vi "Build Command.vi"(8 "Error In":errorcluster, 9 "Field Data":u8[](array[numeric]) format="%02x", 10 "Field Descriptor Byte":u8=117 format="%02x", 11 "Data Set":T1=enum."NAV") -> (0 "Error Out":errorcluster, 3 "Command":u8[](array[numeric]) format="%02x")   [LabVIEW 2011]
doc: "This VI builds Hex commands for the Microstrain 3DM GX3-45 \n\nSee Microstrain Communications Protocol guide for further details."
uses:
  Controls/Desciptor Set Byte.ctl
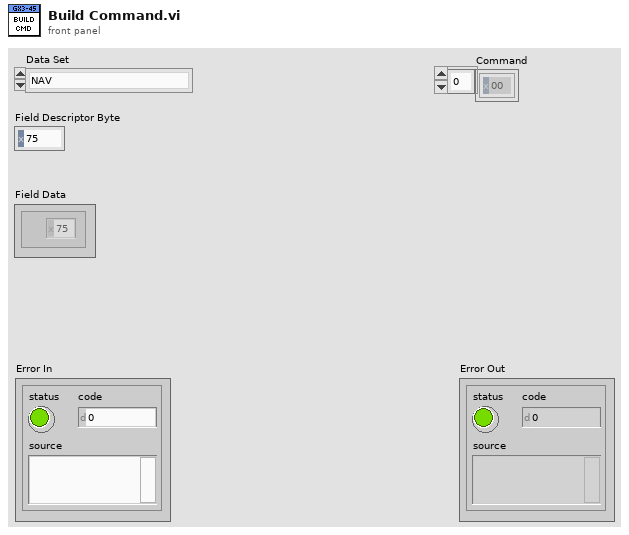
[diagram p1: front panel]
types:
  T1 = typedef "Desciptor Set Byte.ctl" = enum16{"Base Command Set", "3DM Command Set", "Navigation Filter Command Set", "System Command Set", "AHRS", "GPS", "NAV"}
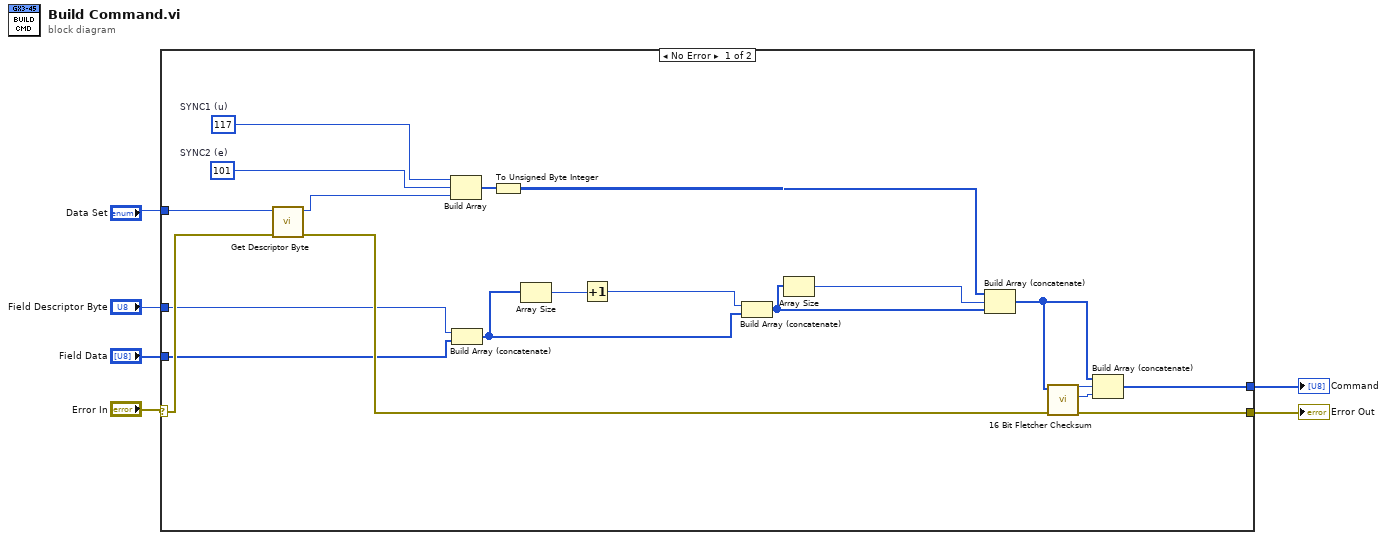
[diagram p0: block diagram]
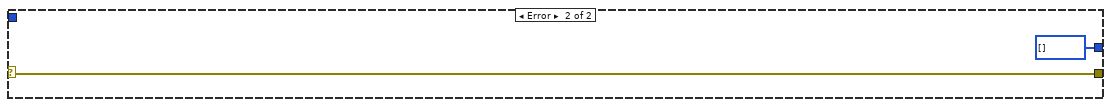
[diagram p2: hidden frame]
diagram:
  n1 = case shown="No Error" "Error In" {
    selector: "Error In" -> [w12 w28]
    tunnel: [w13 w28] -> w6
    tunnel: "Data Set" -> [w10 _]
    tunnel: "Field Descriptor Byte" -> [w9 _]
    tunnel: "Field Data" -> [w8 _]
    tunnel: [w7 i32[] []] -> w1
    frame No Error {
      w25 = u8 101  # SYNC2 (e)
      w26 = u8 117  # SYNC1 (u)
      n2 = call "Get Descriptor Byte.vi"("Error In"=w12, "Data Set"=w10) -> ("Error Out"=w11:errorcluster, "Desciptor Byte"=w24:u8)  [unwired: 8 in]
      n3 = Build Array(w26, w25, w24) -> (w17:u8[])
      n4 = Build Array (concatenate)(w9, w8) -> (w22:u8[])
      n5 = To Unsigned Byte Integer(number=w17) -> (unsigned 8bit integer=w16:u8[])
      n6 = Array Size(array=w22) -> (size(s)=w23:i32)
      n7 = Increment(x=w23) -> (x+1=w21:i32)
      n8 = Build Array (concatenate)(w21, w22) -> (w20:i32[])
      n9 = Array Size(array=w20) -> (size(s)=w19:i32)
      n10 = Build Array (concatenate)(w16, w19, w20) -> (w18:i32[])
      n11 = call "16 Bit Fletcher Checksum.vi"("Error In"=w11, "Input Array"=w18) -> ("Error Out"=w13:errorcluster, "B (LSB)"=w15:u8, "A (MSB)"=w14:u8)  [unwired: 7 in]
      n12 = Build Array (concatenate)(w18, w14, w15) -> (w7:i32[])
    }
    frame Error {
    }
  }
  "Error Out" <- w6
  "Command" <- w1
